vi "Network Stream.vi"(11 "Queue Ref":T1) -> ()   [LabVIEW 2022 SP3]
uses:
  Controls/All Queue.ctl
  Controls/Network Stream.ctl
  Controls/All Loop Status.ctl
  Global 1.vi
panel:
  out "x-y":u32
  out "error out":errorcluster
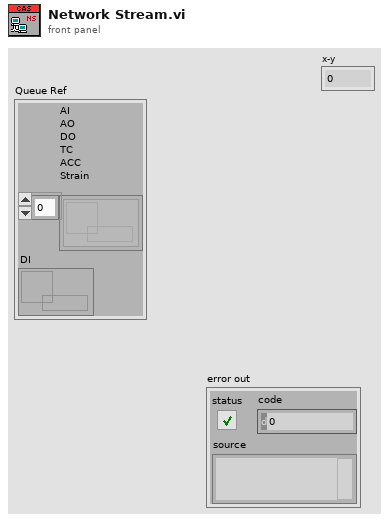
[diagram p1: front panel]
types:
  T1 = typedef "All Queue.ctl" = cluster{"AI\nAO\nDO\nTC\nACC\nStrain":refnum<queue>[], "DI":refnum<queue>}
  T2 = cluster{"in progress?":bool, "Queue Ref ":T1, "writer name":refnum<k21>, "Reader name":refnum<k21>}
  T3 = typedef "Network Stream.ctl" = enum16{"Initialize", "Wait For connection", "Wait for Data", "Exit", "Close Connection"}
  T4 = typedef "All Loop Status.ctl" = enum16{"AI", "AO", "DI", "DO", "TC", "Strain", "ACC", "RT", "Log", "Seq"}
  T5 = enum16{"Init", "Read 'All'", "Read 'n'", "Read '1'", "Write '1'", "Write 'n'", "Write 'All'"}
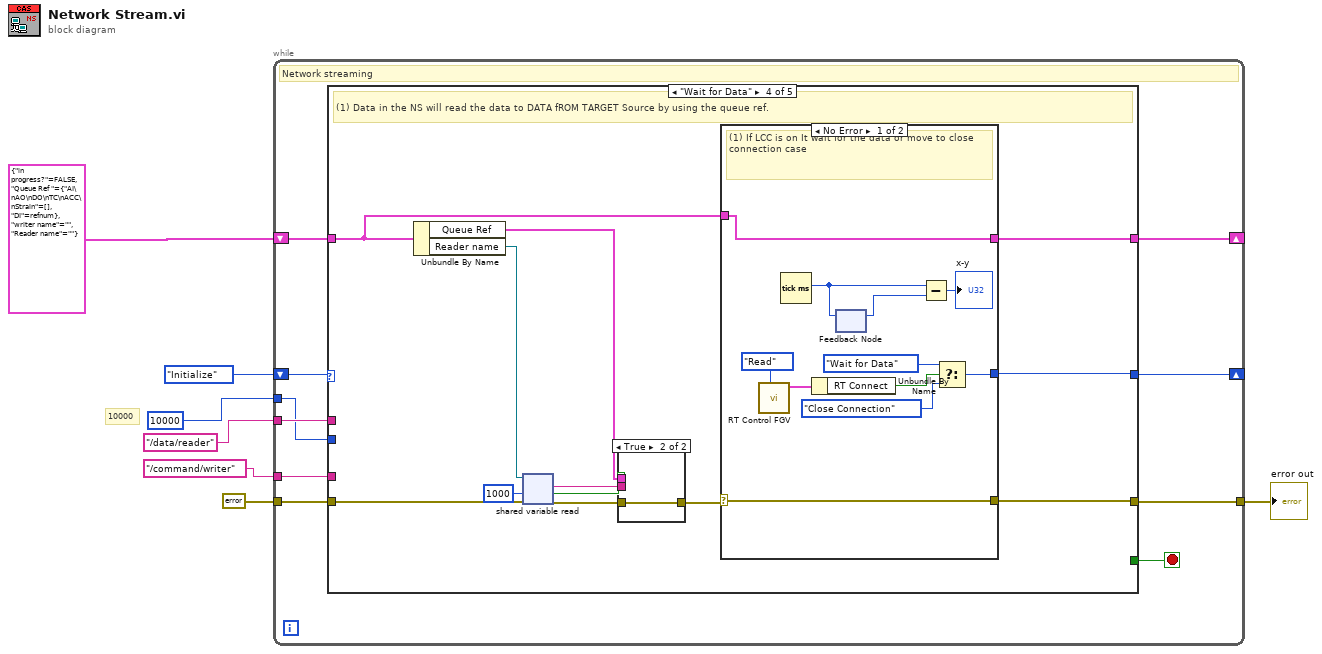
[diagram p0: block diagram]
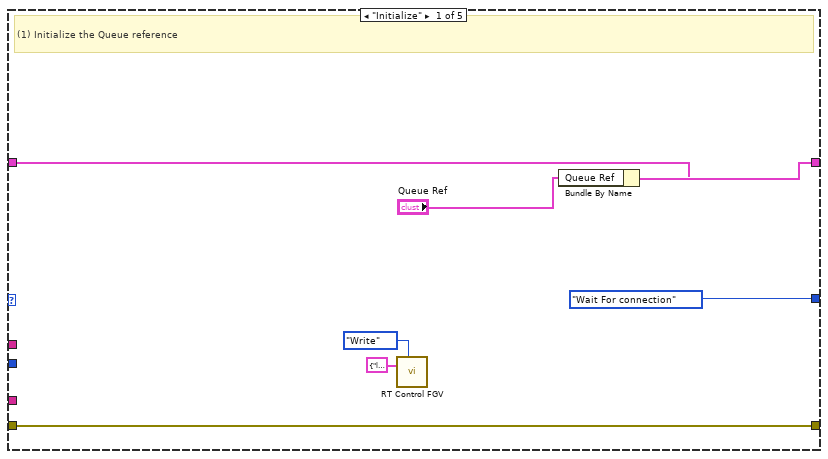
[diagram p2: hidden frame]
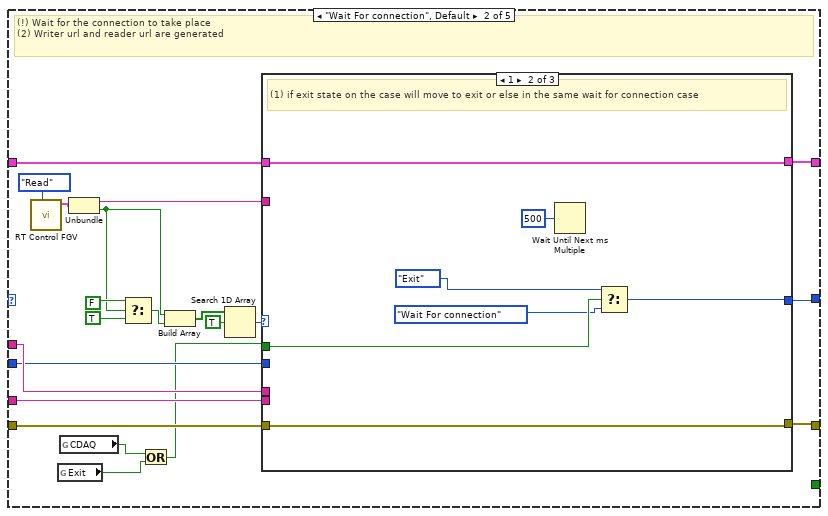
[diagram p3: hidden frame]
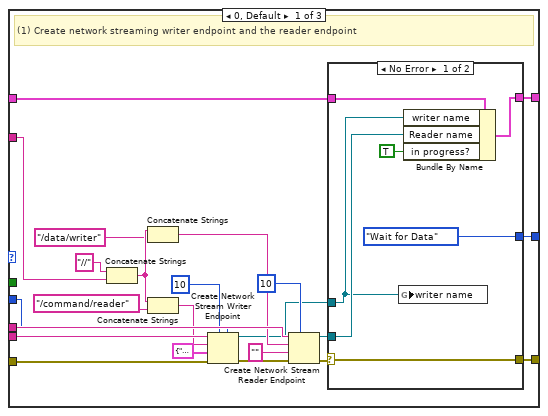
[diagram p4: hidden frame]
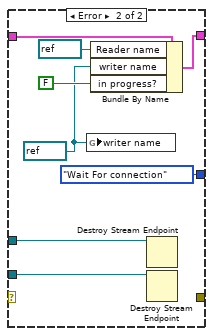
[diagram p5: hidden frame]
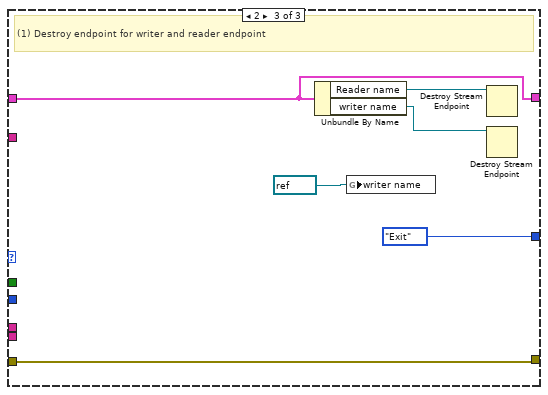
[diagram p6: hidden frame]
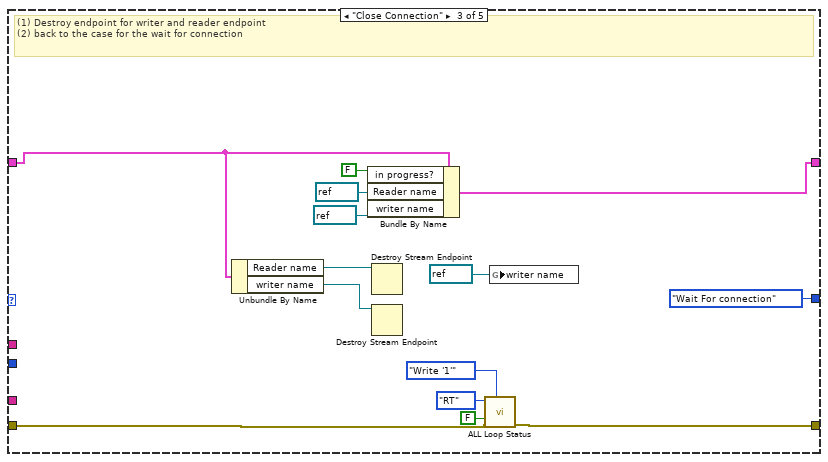
[diagram p7: hidden frame]
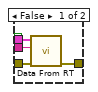
[diagram p8: hidden frame]
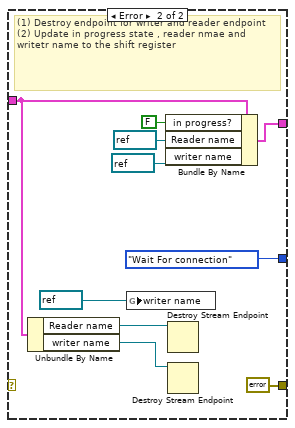
[diagram p9: hidden frame]
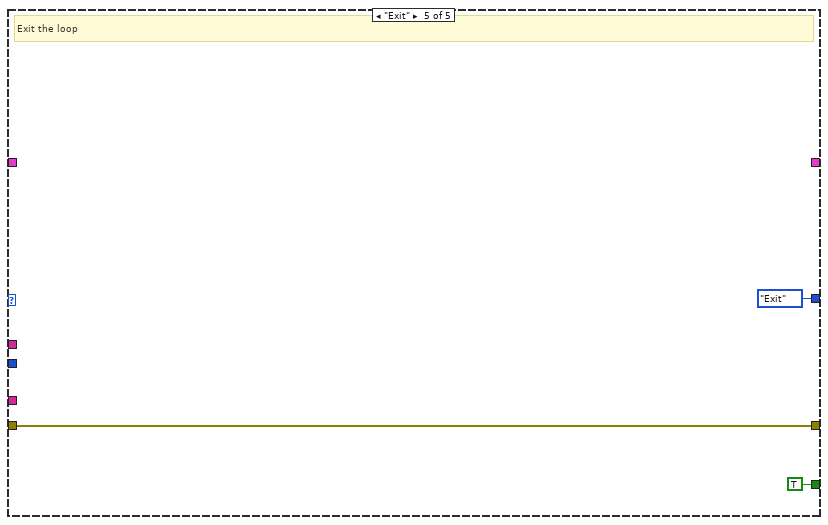
[diagram p10: hidden frame]
diagram:
  # "10000"
  n1 = while {
    shift-right: [w13] -> _
    shift-left: Network_Stream."Initialize" -> [w17]
    shift-right: [w15] -> _
    shift-left: T2 {"in progress?"=FALSE, "Queue Ref "={"AI\nAO\nDO\nTC\nACC\nStrain"=[], "DI"=refnum}, "writer name"="", "Reader name"=""} -> [w8]
    tunnel: errorcluster {"status"=FALSE, "code"=0, "source"=""} ("error in") -> [w14]
    tunnel: [w9] -> w5
    tunnel: "/command/writer" ("writer name") -> [w12]
    tunnel: "/data/reader" ("writer name") -> [w11]
    tunnel: 10000 ("timeout in ms (-1)") -> [w10]
    stop <- w16 stop-if-true
    # "Network streaming"
    n2 = case shown="\"Wait for Data\"" w17 {
      tunnel: [_ _ _ _ TRUE] -> w16
      tunnel: w8 -> [w23 w42 w104 w120 _]
      tunnel: [w24 w41 w103 w119 _] -> w15
      tunnel: w14 -> [w22 w45 w101 w122 w149]
      tunnel: [w22 w39 w100 w118 w149] -> w9
      tunnel: [Network_Stream."Wait For connection" w40 Network_Stream."Wait For connection" w121 Network_Stream."Exit"] -> w13
      tunnel: w12 -> [_ w44 _ _ _]
      tunnel: w11 -> [_ w43 _ _ _]
      tunnel: w10 -> [_ w32 _ _ _]
      frame "Initialize" {
        # "(1) Initialize the Queue reference"
        n3 = call "RT Control FGV.vi"("Enum"=enum16{"Read", "Write"}."Write", "RT Ctrl"=cluster{"RT IP":string, "RT Connect":bool} {"RT IP"="localhost", "RT Connect"=FALSE}) -> ()  [unwired: 9 in, 1 out]
        n4 = Bundle By Name(cluster=w23, "Queue Ref"="Queue Ref") -> (w24:T2)
      }
      frame "Wait For connection", Default {
        # "(!) Wait for the connection to take place\n(2) Writer url and reader url are generated"
        n5 = call "RT Control FGV.vi"("Enum"=enum16{"Read", "Write"}."Read") -> ("RT Ctrl out"=w27:cluster{"RT IP":string, "RT Connect":bool})  [unwired: 10 in]
        n6 = global read "Global 1.vi" "Exit"() -> (w30:bool)
        n7 = global read "Global 1.vi" "CDAQ"() -> (w31:bool)
        n8 = Unbundle(w27) -> ("RT IP"=w25:string, "RT Connect"=w26:bool)
        n9 = Select(t=FALSE ("LCC ON/OFF"), s=w26, f=TRUE ("LCC ON/OFF")) -> (s? t:f=w33:bool)
        n10 = Or(x=w31, y=w30) -> (x .or. y?=w29:bool)
        n11 = Build Array(w26, w33) -> (w37:bool[])
        n12 = Search 1D Array(1D array=w37, element=TRUE) -> (index of element=w38:i32)  [unwired: 1 in]
        n13 = case shown="1" w38 {
          tunnel: w45 -> [w68 w89 w93]
          tunnel: w44 -> [w64 _ _]
          tunnel: w43 -> [w63 _ _]
          tunnel: w42 -> [w54 w90 w94]
          tunnel: [w53 w90 w94] -> w41
          tunnel: [w51 w87 Network_Stream."Exit"] -> w40
          tunnel: [w49 w89 w93] -> w39
          tunnel: w32 -> [w48 _ _]
          tunnel: w29 -> [_ w88 _]
          tunnel: w25 -> [w46 _ _]
          frame 0, Default {
            # "(1) Create network streaming writer endpoint and the reader endpoint"
            n14 = Concatenate Strings("//" ("reader url"), w46) -> (w60:string)
            n15 = Concatenate Strings(w60, "/data/writer" ("reader url")) -> (w58:string)
            n16 = Concatenate Strings(w60, "/command/reader" ("reader url")) -> (w57:string)
            n17 = Create Network Stream Writer Endpoint(5:w48, 7:10 ("writer buffer size"), 8:w68, 9:cluster{"Message":string, "Data":variant} {"Message"="", "Data"=variant}, 10:w57, 11:w64) -> (0:w67:errorcluster, 3:w47:refnum<k21>)  [unwired: 1 in]
            n18 = Create Network Stream Reader Endpoint(7:10 ("writer buffer size"), 8:w67, 9:"" ("reader url"), 10:w58, 11:w63) -> (0:w52:errorcluster, 3:w50:refnum<k21>)  [unwired: 2 in]
            n19 = case shown="No Error" w52 {
              selector: w52 -> [w71 _]
              tunnel: w54 -> [w74 w79]
              tunnel: [w75 w80] -> w53
              tunnel: w47 -> [w70 w81]
              tunnel: w50 -> [w72 w83]
              tunnel: [Network_Stream."Wait for Data" Network_Stream."Wait For connection"] -> w51
              tunnel: [w71 _] -> w49
              frame No Error {
                n20 = global write "Global 1.vi" "writer name"(w70) -> ()
                n21 = Bundle By Name(cluster=w74, "writer name"=w70, "Reader name"=w72, "in progress?"=TRUE) -> (w75:T2)
              }
              frame Error {
                w76 = refnum<k21> refnum ("writer name")
                n22 = global write "Global 1.vi" "writer name"(w76) -> ()
                n23 = Bundle By Name(cluster=w79, "Reader name"=refnum<k21> refnum, "writer name"=w76, "in progress?"=FALSE) -> (w80:T2)
                n24 = Destroy Stream Endpoint(11:w81) -> ()  [unwired: 1 in, 1 out]
                n25 = Destroy Stream Endpoint(11:w83) -> ()  [unwired: 1 in, 1 out]
              }
            }
          }
          frame 1 {
            # "(1) if exit state on the case will move to exit or else in the same wait for connection case"
            n26 = Wait Until Next ms Multiple(millisecond multiple=u32 500) -> ()  [unwired: 1 out]
            n27 = Select(t=Network_Stream."Exit", s=w88, f=Network_Stream."Wait For connection") -> (s? t:f=w87:T3)
          }
          frame 2 {
            # "(1) Destroy endpoint for writer and reader endpoint"
            n28 = Unbundle By Name(w94) -> ("Reader name"=w96:refnum<k21>, "writer name"=w95:refnum<k21>)
            n29 = global write "Global 1.vi" "writer name"(refnum<k21> refnum ("writer name")) -> ()
            n30 = Destroy Stream Endpoint(11:w96) -> ()  [unwired: 1 in, 1 out]
            n31 = Destroy Stream Endpoint(11:w95) -> ()  [unwired: 1 in, 1 out]
          }
        }
      }
      frame "Close Connection" {
        # "(1) Destroy endpoint for writer and reader endpoint\n(2) back to the case for the wait for connection"
        n32 = Unbundle By Name(w104) -> ("Reader name"=w109:refnum<k21>, "writer name"=w108:refnum<k21>)
        n33 = Bundle By Name(cluster=w104, "in progress?"=FALSE, "Reader name"=refnum<k21> refnum, "writer name"=refnum<k21> refnum) -> (w103:T2)
        n34 = Destroy Stream Endpoint(11:w109) -> ()  [unwired: 1 in, 1 out]
        n35 = Destroy Stream Endpoint(11:w108) -> ()  [unwired: 1 in, 1 out]
        n36 = call "ALL Loop Status.vi"("Option"=T5."Write '1'", "error in (no error)"=w101, "Status"=FALSE, "Loop"=All_Loop_Status."RT") -> ("error out"=w100:errorcluster)  [unwired: 5 in, 2 out]
        n37 = global write "Global 1.vi" "writer name"(refnum<k21> refnum ("writer name")) -> ()
      }
      frame "Wait for Data" {
        # "(1) Data in the NS will read the data to DATA fROM TARGET Source by using the queue ref."
        n38 = Unbundle By Name(w120) -> ("Queue Ref"=w116:T1, "Reader name"=w117:refnum<k21>)
        n39 = shared-variable-read(w117, w122, 1000 ("timeout ms (-1)")) -> (w114:errorcluster, w111:bool, w115:string)  [unwired: 1 out]
        n40 = case shown="True" w111 {
          tunnel: w116 -> [w126 _]
          tunnel: w115 -> [w125 _]
          tunnel: w114 -> [w124 w127]
          tunnel: [w123 w127] -> w113
          frame False {
            n41 = call "Data From RT.vi"("Queue Ref"=w126, "Data in"=w125, "error in"=w124) -> ("error out"=w123:errorcluster)  [unwired: 7 in]
          }
          frame True {
          }
        }
        n42 = case shown="No Error" w113 {
          selector: w113 -> [w138 _]
          tunnel: [w134 Network_Stream."Wait For connection"] -> w121
          tunnel: w120 -> [w137 w145]
          tunnel: [w137 w144] -> w119
          tunnel: [w138 errorcluster {"status"=FALSE, "code"=0, "source"=""} ("error IO")] -> w118
          frame No Error {
            # "(1) If LCC is on It wait for the data or move to close connection case"
            n43 = call "RT Control FGV.vi"("Enum"=enum16{"Read", "Write"}."Read") -> ("RT Ctrl out"=w132:cluster{"RT IP":string, "RT Connect":bool})  [unwired: 10 in]
            n44 = Tick Count (ms)() -> (millisecond timer value=w129:u32)
            n45 = Unbundle By Name(w132) -> ("RT Connect"=w131:bool)
            n46 = feedback-in #1(w129) -> ()
            n47 = feedback #1() -> (w130:u32)  [unwired: 1 in]
            n48 = Subtract(x=w129, y=w130) -> (x-y=→"x-y":u32)
            n49 = Select(t=Network_Stream."Wait for Data", s=w131, f=Network_Stream."Close Connection") -> (s? t:f=w134:T3)
          }
          frame Error {
            # "(1) Destroy endpoint for writer and reader endpoint\n(2) Update in progress state , reader nmae and writetr name to the shift register"
            n50 = Unbundle By Name(w145) -> ("Reader name"=w147:refnum<k21>, "writer name"=w146:refnum<k21>)
            n51 = global write "Global 1.vi" "writer name"(refnum<k21> refnum ("writer name")) -> ()
            n52 = Bundle By Name(cluster=w145, "in progress?"=FALSE, "Reader name"=refnum<k21> refnum, "writer name"=refnum<k21> refnum) -> (w144:T2)
            n53 = Destroy Stream Endpoint(11:w147) -> ()  [unwired: 1 in, 1 out]
            n54 = Destroy Stream Endpoint(11:w146) -> ()  [unwired: 1 in, 1 out]
          }
        }
      }
      frame "Exit" {
        # "Exit the loop"
      }
    }
  }
  "error out" <- w5
